vi "Save with Header old.vi"(4 "transpose? (no:F)":bool, 5 "format (%.3f)":string, 9 "Header":string, 10 "2D data":dbl[][](array[numeric]) format="%.2f", 11 "file path (dialog if empty)":path) -> (3 "new file path (Not A Path if cancelled)":path)   [LabVIEW 2021]
uses:
  <vilib>/Utility/file.llb/Write To Spreadsheet File (DBL).vi
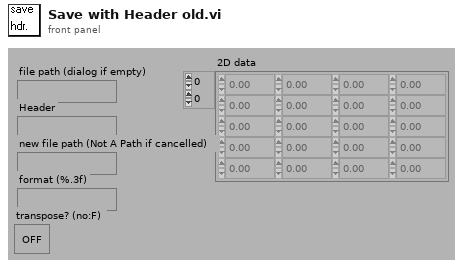
[diagram p1: front panel]
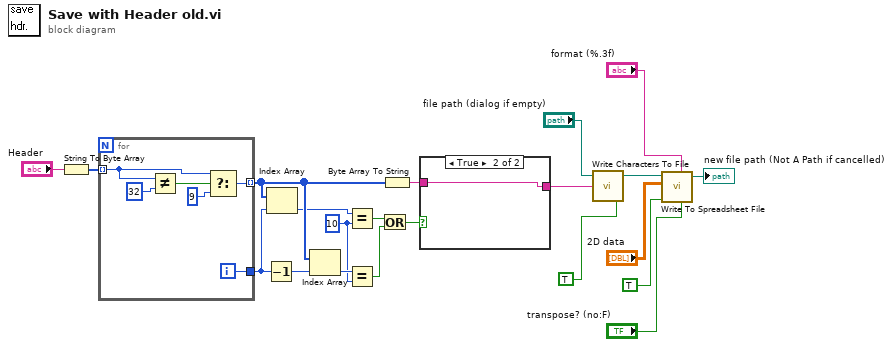
[diagram p0: block diagram]
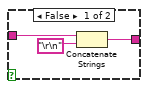
[diagram p2: hidden frame]
diagram:
  w6 = u8 10
  n1 = String To Byte Array(string="Header") -> (unsigned byte array=w11:u8[])
  n2 = for {
    tunnel: w11 -> [w25] mode=indexing
    tunnel: [w23] -> w10 mode=indexing
    tunnel: [w22] -> w1
    i -> [w22]
    n3 = Not Equal?(x=w25, y=u8 32) -> (x != y?=w26:bool)
    n4 = Select(t=w25, s=w26, f=u8 9) -> (s? t:f=w23:u8)
  }
  n5 = Decrement(x=w1) -> (x-1=w9:i32)
  n6 = Index Array(array=w10, index=w1) -> (element=w8:u8)
  n7 = Index Array(array=w10, index=w9) -> (element=w7:u8)
  n8 = Equal?(x=w8, y=w6) -> (x = y?=w5:bool)
  n9 = Equal?(x=w7, y=w6) -> (x = y?=w4:bool)
  n10 = Or(x=w5, y=w4) -> (x .or. y?=w3:bool)
  n11 = Byte Array To String(unsigned byte array=w10) -> (string=w2:string)
  n12 = case shown="True" w3 {
    tunnel: w2 -> [w29 w31]
    tunnel: [w28 w31] -> w12
    frame False {
      n13 = Concatenate Strings(w29, "\r\n") -> (w28:string)
    }
    frame True {
    }
  }
  n14 = call <vilib>:"Write Characters To File.vi"("convert eol? (no:F)"=TRUE, "character string"=w12, "file path (dialog if empty)"="file path (dialog if empty)") -> ("new file path (Not A Path if cancelled)"=w18:path)  [unwired: 1 in, 1 out]
  n15 = call-poly <vilib>:"Write To Spreadsheet File.vi"("transpose? (no:F)"="transpose? (no:F)", "format (%.3f)"="format (%.3f)", "append to file? (new file:F)"=TRUE, "2D data"="2D data", "file path (dialog if empty)"=w18) -> ("new file path (Not A Path if cancelled)"=→"new file path (Not A Path if cancelled)":path)  [unwired: 1 in, 2 out]
